vi "Write.vi"(5 "TDMS File in":refnum<class "File.lvclass">, 8 "error in (no error)":errorcluster, 9 "File Properties":refnum<class "Variant.lvclass">, 10 "Groups":refnum<class "Group.lvclass">[](array[class]), 11 "File Path":path) -> (0 "error out":errorcluster, 3 "TDMS File out":refnum<class "File.lvclass">)   [LabVIEW 2020, in "TDMS.lvlib" / "File.lvclass"]
doc: "Write File Path, Groups and File Properties."
uses:
  File.lvclass
  TDMS Group/Group.lvclass
  PPL/HDH.Data.Generic.lvlibp/Generic Data/Variant/Variant.lvclass
  File.lvclass/File.ctl
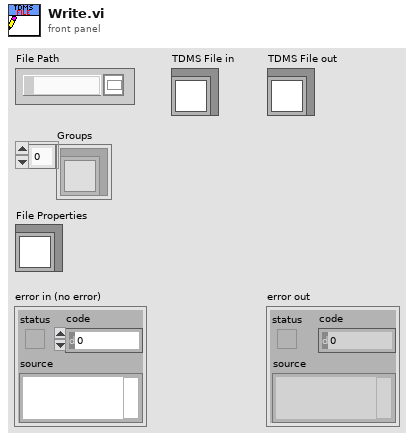
[diagram p1: front panel]
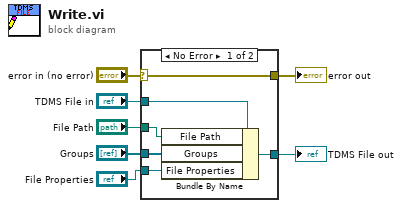
[diagram p0: block diagram]
diagram:
  n1 = case shown="No Error" "error in (no error)" {
    selector: "error in (no error)" -> [w13 w14]
    tunnel: [w13 w14] -> w6
    tunnel: [w11 w15] -> w4
    tunnel: "TDMS File in" -> [w12 w15]
    tunnel: "File Path" -> [w10 _]
    tunnel: "Groups" -> [w9 _]
    tunnel: "File Properties" -> [w8 _]
    frame No Error {
      n2 = Bundle By Name(cluster=w12, "File Path"=w10, "Groups"=w9, "File Properties"=w8) -> (w11:refnum<class "File.lvclass">)
    }
    frame Error {
    }
  }
  "error out" <- w6
  "TDMS File out" <- w4
